vi "Check for Names v2.vi"(0 "New Name":string, 1 "Name List":string[](array[string]), 2 "Empty Plots?":bool[](array[boolean]), 3 "Error In":errorcluster, 4 "Suffix Format String (<Space>%d)":string=" %d") -> (5 "New Name List":string[](array[string]), 6 "New Name":string, 7 "Checked Array":bool[](array[boolean]), 9 "Error Out":errorcluster)   [LabVIEW 2021, in "Strings.lvlib"]
uses:
  Strings.lvlib
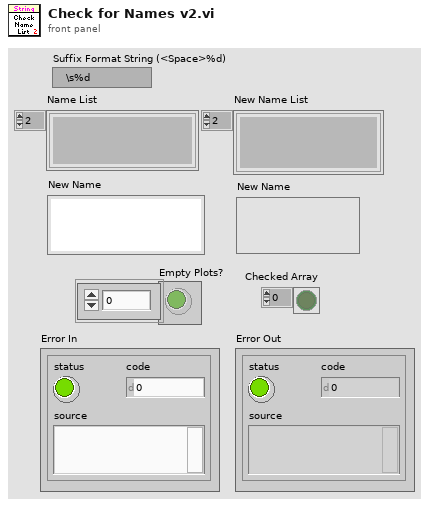
[diagram p1: front panel]
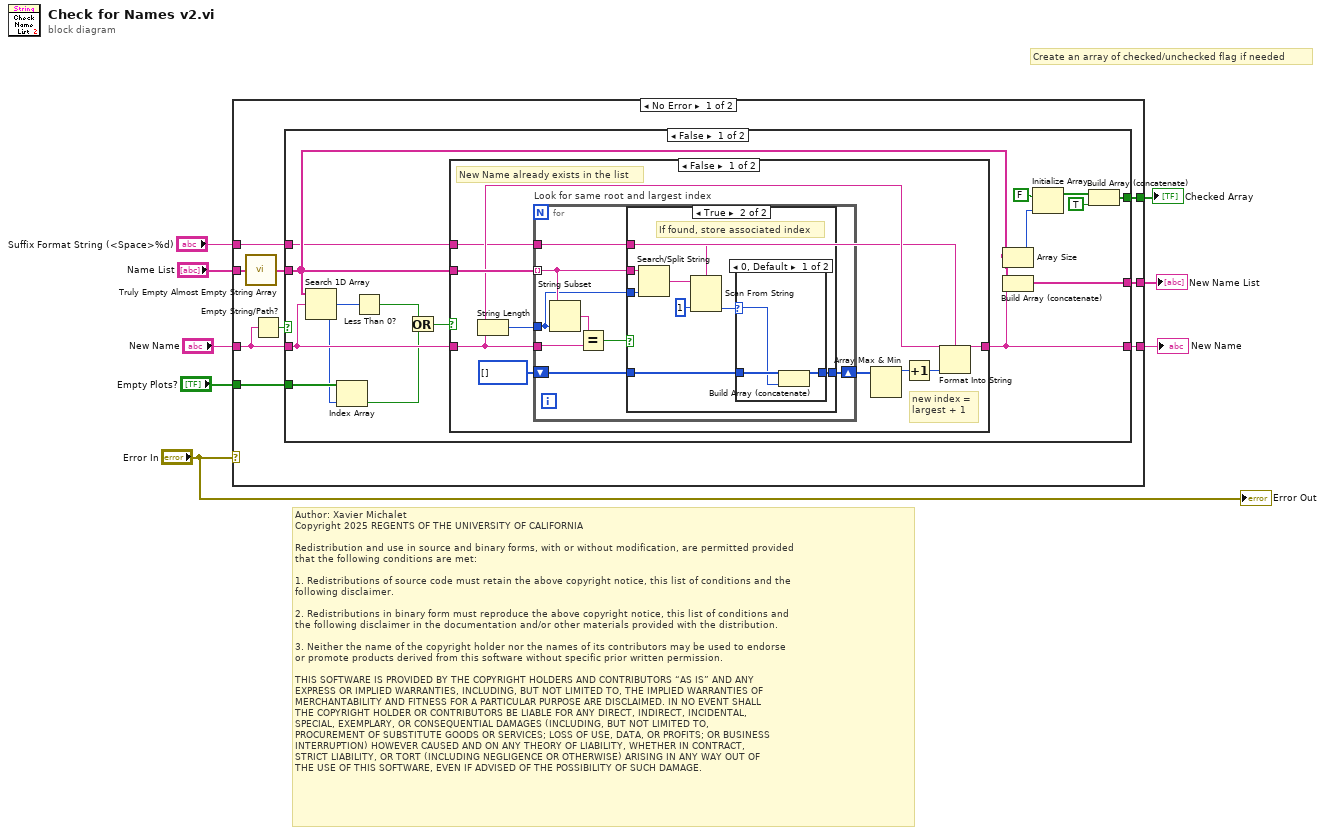
[diagram p0: block diagram]
diagram:
  # "Author: Xavier Michalet\nCopyright 2025 REGENTS OF THE UNIVERSITY OF CALIFORNIA\n\nRedistribution and use in source and binary forms, with or without modification, are permitted provided\nthat the following conditions are met:\n\n1. Redistributions of source code must retain the above copyright notice, this list of conditions and the\nfollowing disclaimer.\n\n2. Redistributions in binary form must reproduce the above copyright notice, this list of conditions and\nthe following disclaimer in the documentation and/or other materials provided with the distribution.\n\n3. Neither the name of the copyright holder nor the names of its contributors may be used to endorse \nor promote products derived from this software without specific prior written permission.\n\nTHIS SOFTWARE IS PROVIDED BY THE COPYRIGHT HOLDERS AND CONTRIBUTORS “AS IS” AND ANY \nEXPRESS OR IMPLIED WARRANTIES, INCLUDING, BUT NOT LIMITED TO, THE IMPLIED WARRANTIES OF\nMERCHANTABILITY AND FITNESS FOR A PARTICULAR PURPOSE ARE DISCLAIMED. IN NO EVENT SHALL\nTHE COPYRIGHT HOLDER OR CONTRIBUTORS BE LIABLE FOR ANY DIRECT, INDIRECT, INCIDENTAL, \nSPECIAL, EXEMPLARY, OR CONSEQUENTIAL DAMAGES (INCLUDING, BUT NOT LIMITED TO, \nPROCUREMENT OF SUBSTITUTE GOODS OR SERVICES; LOSS OF USE, DATA, OR PROFITS; OR BUSINESS\nINTERRUPTION) HOWEVER CAUSED AND ON ANY THEORY OF LIABILITY, WHETHER IN CONTRACT, \nSTRICT LIABILITY, OR TORT (INCLUDING NEGLIGENCE OR OTHERWISE) ARISING IN ANY WAY OUT OF\nTHE USE OF THIS SOFTWARE, EVEN IF ADVISED OF THE POSSIBILITY OF SUCH DAMAGE."
  # "Create an array of checked/unchecked flag if needed"
  n1 = case shown="No Error" "Error In" {
    tunnel: [w17 w66] -> w8
    tunnel: [w16 w67] -> w7
    tunnel: [w15 _] -> w6
    tunnel: "Name List" -> [w9 w67]
    tunnel: "New Name" -> [w14 w66]
    tunnel: "Empty Plots?" -> [w12 _]
    tunnel: "Suffix Format String (<Space>%d)" -> [w11 _]
    frame No Error {
      n2 = call "Truly Empty Almost Empty String Array.vi"("String Array"=w9) -> ("String Array"=w10:string[])  [unwired: 14 in]
      n3 = Empty String/Path?(string/path=w14) -> (empty?=w13:bool)
      n4 = case shown="False" w13 {
        tunnel: [w32 w64] -> w17
        tunnel: [w31 w65] -> w16
        tunnel: [w26 _] -> w15
        tunnel: w10 -> [w25 w65]
        tunnel: w14 -> [w24 w64]
        tunnel: w12 -> [w23 _]
        tunnel: w11 -> [w18 _]
        frame False {
          n5 = Search 1D Array(1D array=w25, element=w24) -> (index of element=w22:i32)  [unwired: 1 in]
          n6 = Index Array(array=w23, index=w22) -> (element=w20:bool)
          n7 = Less Than 0?(x=w22) -> (x < 0?=w21:bool)
          n8 = Or(x=w21, y=w20) -> (x .or. y?=w19:bool)
          n9 = case shown="False" w19 {
            tunnel: w24 -> [w34 w63]
            tunnel: [w36 w63] -> w32
            tunnel: w25 -> [w41 _]
            tunnel: w18 -> [w33 _]
            frame False {
              # "new index =\nlargest + 1"
              # "New Name already exists in the list"
              n10 = String Length(string=w34) -> (length=w35:i32)
              n11 = for "Look for same root and largest index" {
                tunnel: w41 -> [w44] mode=indexing
                tunnel: w34 -> [w46]
                shift-right: [w48] -> w39
                shift-left: i32[] [] -> [w49]
                tunnel: w35 -> [w43]
                tunnel: w33 -> [w42]
                n12 = String Subset(string=w44, length (rest)=w43) -> (substring=w47:string)  [unwired: 1 in]
                n13 = Equal?(x=w47, y=w46) -> (x = y?=w45:bool)
                n14 = case shown="True" w45 {
                  tunnel: w49 -> [w50 w57]
                  tunnel: [w50 w56] -> w48
                  tunnel: w44 -> [_ w55]
                  tunnel: w43 -> [_ w54]
                  tunnel: w42 -> [_ w51]
                  frame False {
                  }
                  frame True {
                    # "If found, store associated index"
                    n15 = Search/Split String(string=w55, offset (0)=w54) -> (match + rest of string=w53:string)  [unwired: 1 in, 2 out]
                    n16 = Scan From String(format string=w51, input string=w53, default 1=1 ("Default Value 1")) -> (output 1=w52:i32)  [unwired: 2 in, 3 out]
                    n17 = case shown="0, Default" w52 {
                      selector: w52 -> [w59 _]
                      tunnel: w57 -> [w61 w62]
                      tunnel: [w60 w62] -> w56
                      frame 0, Default {
                        n18 = Build Array (concatenate)(w61, w59) -> (w60:i32[])
                      }
                      frame -1 {
                        # "not an index"
                      }
                    }
                  }
                }
              }
              n19 = Array Max & Min(array=w39) -> (max value=w38:i32)  [unwired: 3 out]
              n20 = Increment(x=w38) -> (x+1=w37:i32)
              n21 = Format Into String(format string=w33, initial string=w34, w37) -> (resulting string=w36:string)  [unwired: 1 in, 1 out]
            }
            frame True {
              # "New Name does not conflict with any existing ones\nor it is because the plot is empty"
            }
          }
          n22 = Array Size(array=w25) -> (size(s)=w30:i32)
          n23 = Build Array (concatenate)(w25, w32) -> (w31:string[])
          n24 = Initialize Array(FALSE, w30) -> (w28:bool[])
          n25 = Build Array (concatenate)(w28, TRUE ("Input Element")) -> (w26:bool[])
        }
        frame True {
        }
      }
    }
    frame Error {
    }
  }
  "New Name" <- w8
  "New Name List" <- w7
  "Checked Array" <- w6
  "Error Out" <- "Error In"
